vi "Lire Exchanges.vi"(11 "Portfolio en entrée":refnum<class "Portfolio.lvclass">) -> (2 "Exchanges.lvclass":refnum<class "Exchanges.lvclass">, 3 "Portfolio en sortie":refnum<class "Portfolio.lvclass">)   [LabVIEW 2012, in "Portfolio.lvclass"]
uses:
  Portfolio.lvclass
  Exchanges/Exchanges.lvclass
  Portfolio.lvclass/Portfolio.ctl
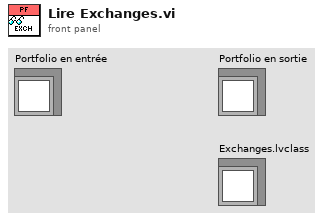
[diagram p1: front panel]
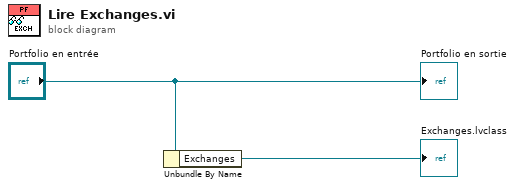
[diagram p0: block diagram]
diagram:
  n1 = Unbundle By Name("Portfolio en entrée") -> ("Exchanges"=→"Exchanges.lvclass":refnum<class "Exchanges.lvclass">)
  "Portfolio en sortie" <- "Portfolio en entrée"
